vi "Load Config.vi"(8 "error in (no error)":errorcluster, 10 "Promise":refnum<class "Promise.lvclass">, 11 "VolatusConfig in":refnum<class "VolatusConfigManager.lvclass">) -> (0 "error out":errorcluster, 3 "VolatusConfig out":refnum<class "VolatusConfigManager.lvclass">)   [LabVIEW 2020, in "Volatus.lvlib" / "VolatusConfigManager.lvclass"]
uses:
  VolatusConfigManager.lvclass
  C:/dev/lv20CE/relink/lv-volatus/Volatus/Task/Task.lvclass
  lv-promises/Promises/Promise/Promise.lvclass
  VolatusConfigManager.lvclass/VolatusConfigManager.ctl
  VolatusNodeValue/VolatusNodeValue.lvclass/VolatusNodeValue.ctl
  Task/Task.lvclass/Task.ctl
  VolatusAPI/VolatusAPI.lvclass/VolatusAPI.ctl
  Event API/EventAPI.lvclass/EventAPI.ctl
  EventHandler Messages/Handle Event Msg/Handle Event Msg.lvclass/Handle Event Msg.ctl
  <vilib>/ActorFramework/Message Enqueuer/Message Enqueuer.lvclass/Message Enqueuer.ctl
  EventHandler Messages/Handle Event Msg/Send Handle Event.vi
  <vilib>/ActorFramework/Message Enqueuer/Enqueue.vi
  VolatusNodeValue/VolatusNodeValue.lvclass
  C:/dev/lv20CE/relink/lv-promises/Promises/Value/Value.lvclass
  EventHandler Messages/Handle Event Msg/Handle Event Msg.lvclass
  C:/Program Files (x86)/National Instruments/LabVIEW 2020/vi.lib/ActorFramework/Message/Message.lvclass
  <vilib>/ActorFramework/Message Priority Queue/Priority Enqueue.vi
  Task/Task.lvclass
  VolatusConfig/VolatusConfig.lvlib
  VolatusConfig/VolatusConfig/VolatusConfig.lvclass
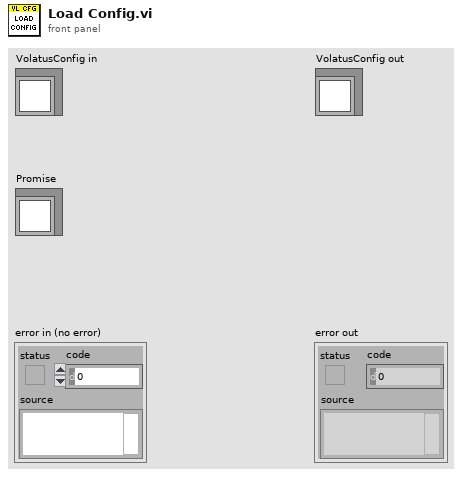
[diagram p1: front panel]
types:
  T1 = typedef "VolatusConfig.lvlib/Config Format.ctl" = enum16{"JSON", "INI", "SQLite"}
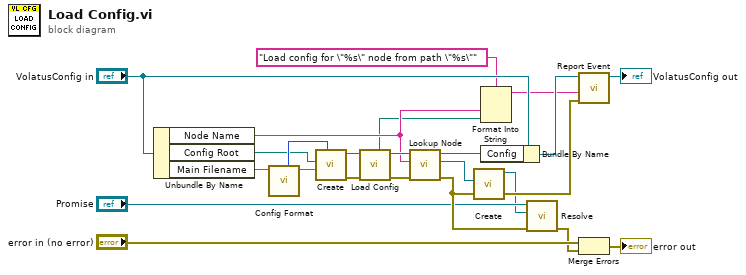
[diagram p0: block diagram]
diagram:
  n1 = Unbundle By Name("VolatusConfig in") -> ("Node Name"=w4:string, "Config Root"=w14:path, "Main Filename"=w15:string)
  n2 = call "Config Format.vi"("Filename"=w15) -> ("filename without extension"=w20:string, "Format"=w21:T1)  [unwired: 9 in]
  n3 = call "Create.vi"("Main Format"=w21, "Main Filename"=w20, "Config Root"=w14) -> ("error out"=w19:errorcluster, "VolatusConfig out"=w17:refnum<class "VolatusConfig.lvclass">)  [unwired: 7 in]
  n4 = call "Load Config.vi"("error in (no error)"=w19, "VolatusConfig in"=w17) -> ("error out"=w18:errorcluster, "VolatusConfig out"=w16:refnum<class "VolatusConfig.lvclass">, "Config Path"=w3:path)  [unwired: 7 in]
  n5 = call "Lookup Node.vi"("error in (no error)"=w18, "Node Name"=w4, "VolatusConfig in"=w16) -> ("error out"=w23:errorcluster, "Node"=w12:refnum<class "Node.lvclass">, "VolatusConfig out"=w13:refnum<class "VolatusConfig.lvclass">)  [unwired: 6 in]
  n6 = call "Create.vi"("Node"=w12) -> ("VolatusNodeValue out"=w10:refnum<class "VolatusNodeValue.lvclass">)  [unwired: 10 in]
  n7 = Format Into String(format string="Load config for \"%s\" node from path \"%s\"", w4, w3) -> (resulting string=w2:string)  [unwired: 2 in, 1 out]
  n8 = Bundle By Name(cluster="VolatusConfig in", "Config"=w13) -> (w7:refnum<class "VolatusConfigManager.lvclass">)
  n9 = call "Resolve.vi"("error in (no error)"=w23, "Result"=w10, "Promise in"="Promise") -> ("error out"=w1:errorcluster)  [unwired: 7 in, 1 out]
  n10 = call "Report Event.vi"("error in (no error)"=w23, "Message"=w2, "Task in"=w7) -> ("Task out"=→"VolatusConfig out":refnum<class "VolatusConfigManager.lvclass">)  [unwired: 7 in, 1 out]
  n11 = Merge Errors("error in (no error)", w1) -> (→"error out":errorcluster)
